vi "To JSON Tree.vi"(8 "error in (no error)":errorcluster, 11 "Request in":refnum<class "Request.lvclass">) -> (0 "error out":errorcluster, 2 "JSON Tree Out":variant, 3 "Request out":refnum<class "Request.lvclass">)   [LabVIEW 2015, in "Request.lvclass"]
uses:
  Request.lvclass
  Request.lvclass/Request.ctl
  <vilib>/NI/i3 JSON/JSON Generation/Create Value Files/Create Value - Object.vi
  has params.vi
  <vilib>/NI/i3 JSON/JSON Generation/Add Object Parameter Files/Add Object Parameter - String.vi
  <vilib>/NI/i3 JSON/JSON Generation/Add Object Parameter Files/Add Object Parameter - Known Type.vi
  id/id.lvclass
  params/params.lvclass
  <vilib>/NI/i3 JSON/i3-json.lvlib
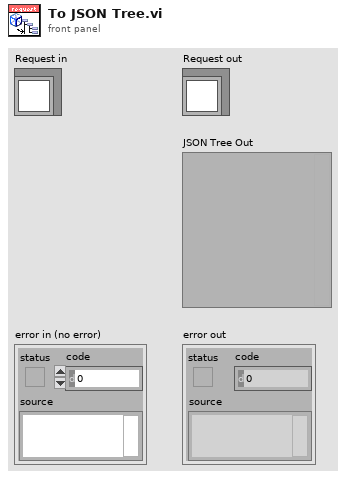
[diagram p1: front panel]
types:
  T1 = typedef "i3-json.lvlib/JSON Type.ctl" = enum8{"JSON Compatible", "JSON Array", "JSON Object", "JSON Null", "Double", "String", "Boolean", "Unknown"}
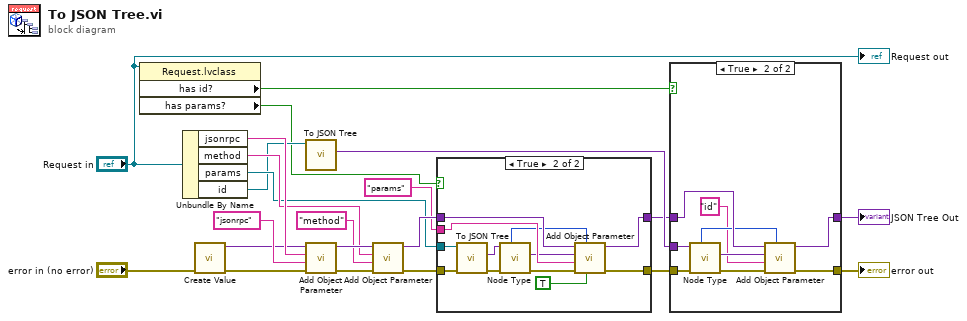
[diagram p0: block diagram]
diagram:
  n1 = property class="Request.lvclass"(reference="Request in") -> ("has id?"=w4:bool, "has params?"=w1:bool)  [unwired: 1 in, 2 out]
  n2 = Unbundle By Name("Request in") -> ("jsonrpc"=w22:string, "method"=w17:string, "params"=w12:refnum<class "params.lvclass">, "id"=w9:refnum<class "id.lvclass">)
  n3 = call-poly <vilib>:"Create Value.vi"("error in (no error)"="error in (no error)") -> ("error out"=w19:errorcluster, "JSON Tree"=w20:variant)  [unwired: 9 in]
  n4 = call-dynamic "To JSON Tree.vi"("id in"=w9) -> ("JSON Tree Out"=w8:variant)  [unwired: 8 in, 2 out]
  n5 = call-poly <vilib>:"Add Object Parameter.vi"("error in (no error)"=w19, "Name"="jsonrpc", "String"=w22, "JSON Tree in (JSON Object)"=w20) -> ("error out"=w10:errorcluster, "JSON Tree out (JSON Object)"=w18:variant)  [unwired: 6 in]
  n6 = call-poly <vilib>:"Add Object Parameter.vi"("error in (no error)"=w10, "Name"="method", "String"=w17, "JSON Tree in (JSON Object)"=w18) -> ("error out"=w14:errorcluster, "JSON Tree out (JSON Object)"=w15:variant)  [unwired: 6 in]
  n7 = case shown="True" w1 {
    tunnel: w15 -> [w23 w36]
    tunnel: w14 -> [w24 w28]
    tunnel: "params" ("Name") -> [_ w35]
    tunnel: w12 -> [_ w34]
    tunnel: [w23 w33] -> w7
    tunnel: [w24 w32] -> w3
    frame False {
    }
    frame True {
      n8 = call-dynamic "To JSON Tree.vi"("error in (no error)"=w28, "params in"=w34) -> ("error out"=w27:errorcluster, "JSON Tree Out"=w31:variant)  [unwired: 7 in, 1 out]
      n9 = call <vilib>:"Node Type.vi"("error in (no error)"=w27, "JSON Tree In"=w31) -> ("error out"=w26:errorcluster, "Value"=w29:variant, "JSON Type"=w30:T1)  [unwired: 5 in, 2 out]
      n10 = call-poly <vilib>:"Add Object Parameter.vi"("Add Parameter as JSON Tree?"=TRUE, "JSON Type"=w30, "error in (no error)"=w26, "Name"=w35, "Value"=w29, "JSON Tree in (JSON Object)"=w36) -> ("error out"=w32:errorcluster, "JSON Tree out (JSON Object)"=w33:variant)  [unwired: 4 in]
    }
  }
  n11 = case shown="True" w4 {
    tunnel: w8 -> [_ w47]
    tunnel: w7 -> [w38 w45]
    tunnel: [w38 w44] -> w6
    tunnel: w3 -> [w37 w41]
    tunnel: [w37 w39] -> w2
    frame False {
    }
    frame True {
      n12 = call <vilib>:"Node Type.vi"("error in (no error)"=w41, "JSON Tree In"=w47) -> ("error out"=w40:errorcluster, "Value"=w46:variant, "JSON Type"=w43:T1)  [unwired: 5 in, 2 out]
      n13 = call-poly <vilib>:"Add Object Parameter.vi"("JSON Type"=w43, "error in (no error)"=w40, "Name"="id", "Value"=w46, "JSON Tree in (JSON Object)"=w45) -> ("error out"=w39:errorcluster, "JSON Tree out (JSON Object)"=w44:variant)  [unwired: 5 in]
    }
  }
  "error out" <- w2
  "JSON Tree Out" <- w6
  "Request out" <- "Request in"
